vi "Bolhas.vi"() -> ()   [LabVIEW 2019]
panel:
  out "Boolean 5":bool
  out "Boolean 4":bool
  out "Boolean 3":bool
  out "Boolean 2":bool
  out "Boolean":bool
  in  "Stop Button":bool
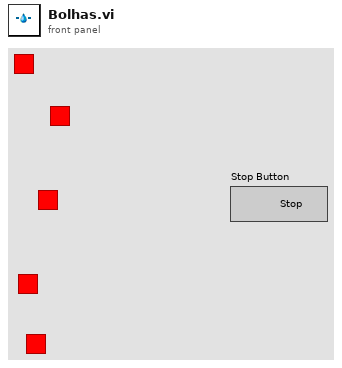
[diagram p1: front panel]
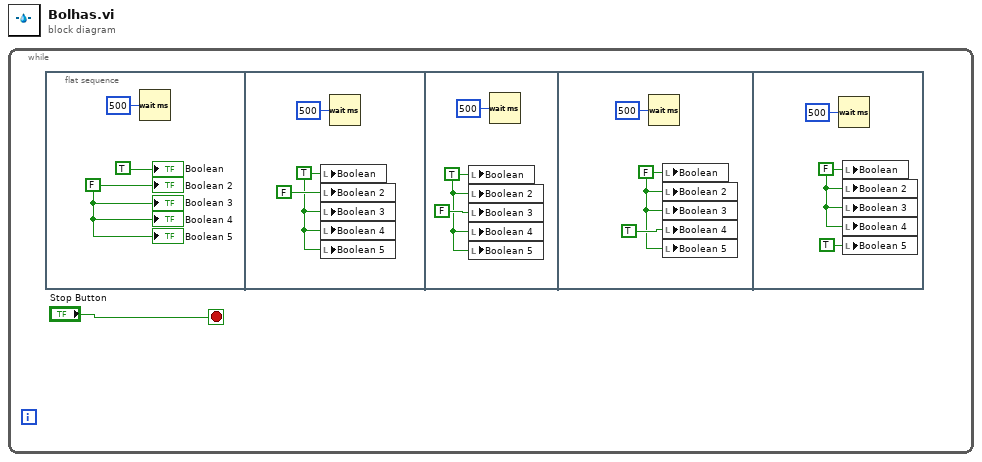
[diagram p0: block diagram]
diagram:
  n1 = while {
    stop <- "Stop Button" stop-if-true
    n2 = flat-sequence {
      frame #0 {
        w2 = FALSE ("Boolean 2")
        n3 = Wait (ms)(milliseconds to wait=u32 500) -> ()  [unwired: 1 out]
        "Boolean" <- TRUE ("Boolean")
        "Boolean 2" <- w2
        "Boolean 5" <- w2
        "Boolean 4" <- w2
        "Boolean 3" <- w2
      }
      frame #1 {
        w5 = TRUE ("Boolean")
        n4 = local write "Boolean"(w5) -> ()
        n5 = local write "Boolean 2"(FALSE ("Boolean 4")) -> ()
        n6 = local write "Boolean 3"(w5) -> ()
        n7 = local write "Boolean 4"(w5) -> ()
        n8 = local write "Boolean 5"(w5) -> ()
        n9 = Wait (ms)(milliseconds to wait=u32 500) -> ()  [unwired: 1 out]
      }
      frame #2 {
        w8 = TRUE ("Boolean")
        n10 = local write "Boolean"(w8) -> ()
        n11 = local write "Boolean 2"(w8) -> ()
        n12 = local write "Boolean 3"(FALSE ("Boolean 5")) -> ()
        n13 = local write "Boolean 4"(w8) -> ()
        n14 = local write "Boolean 5"(w8) -> ()
        n15 = Wait (ms)(milliseconds to wait=u32 500) -> ()  [unwired: 1 out]
      }
      frame #3 {
        w11 = FALSE ("Boolean")
        n16 = Wait (ms)(milliseconds to wait=u32 500) -> ()  [unwired: 1 out]
        n17 = local write "Boolean"(w11) -> ()
        n18 = local write "Boolean 2"(w11) -> ()
        n19 = local write "Boolean 3"(w11) -> ()
        n20 = local write "Boolean 4"(TRUE ("Boolean 2")) -> ()
        n21 = local write "Boolean 5"(w11) -> ()
      }
      frame #4 {
        w14 = FALSE ("Boolean")
        n22 = Wait (ms)(milliseconds to wait=u32 500) -> ()  [unwired: 1 out]
        n23 = local write "Boolean"(w14) -> ()
        n24 = local write "Boolean 2"(w14) -> ()
        n25 = local write "Boolean 3"(w14) -> ()
        n26 = local write "Boolean 4"(w14) -> ()
        n27 = local write "Boolean 5"(TRUE ("Boolean")) -> ()
      }
    }
  }
